vi "U6 Four 32-bit Frequency Measurements.vi"() -> ()   [LabVIEW 2021]
panel:
  out "Frequency (FIO3)":dbl format="%.2f"
  out "Period (FIO3)":dbl format="%.6f"
  out "Frequency (FIO2)":dbl format="%.2f"
  out "Period (FIO2)":dbl format="%.6f"
  in  "DeviceType":u16(ring)=1 items=["LJ_dtU3", "LJ_dtU6", "LJ_dtUE9"]
  out "Frequency (FIO1)":dbl format="%.2f"
  out "Period (FIO1)":dbl format="%.6f"
  out "Iteration":i32
  out "Frequency (FIO0)":dbl format="%.2f"
  out "Period (FIO0)":dbl format="%.6f"
  in  "error in":errorcluster
  in  "ConnectionType":u16(ring) items=["LJ_ctUSB", "LJ_ctETHERNET"]
  in  "Address":string="1"
  in  "FirstFound":bool=TRUE
  in  "stop":bool
  out "error out":errorcluster
  out "Error Message":string
  # "Each iteration, this VI measures the frequency on FIO0-FIO3 using timer mode 2 (32-bit\nperiod measurement).\n\nTested with UD V3.18 and U6 firmware V1.13."
  # "seconds"
  # "seconds"
  # "seconds"
  # "seconds"
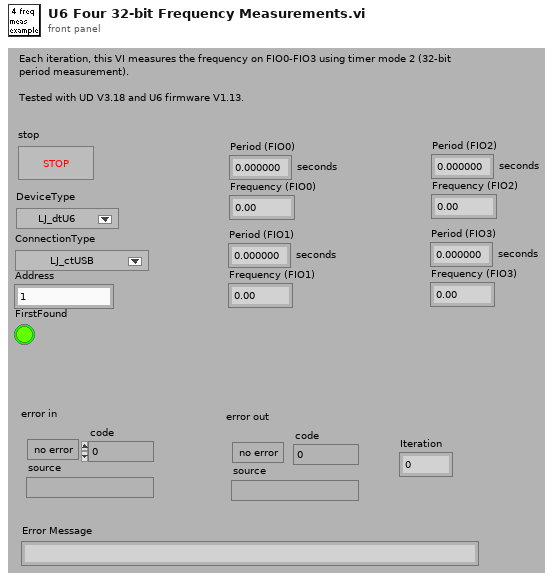
[diagram p1: front panel]
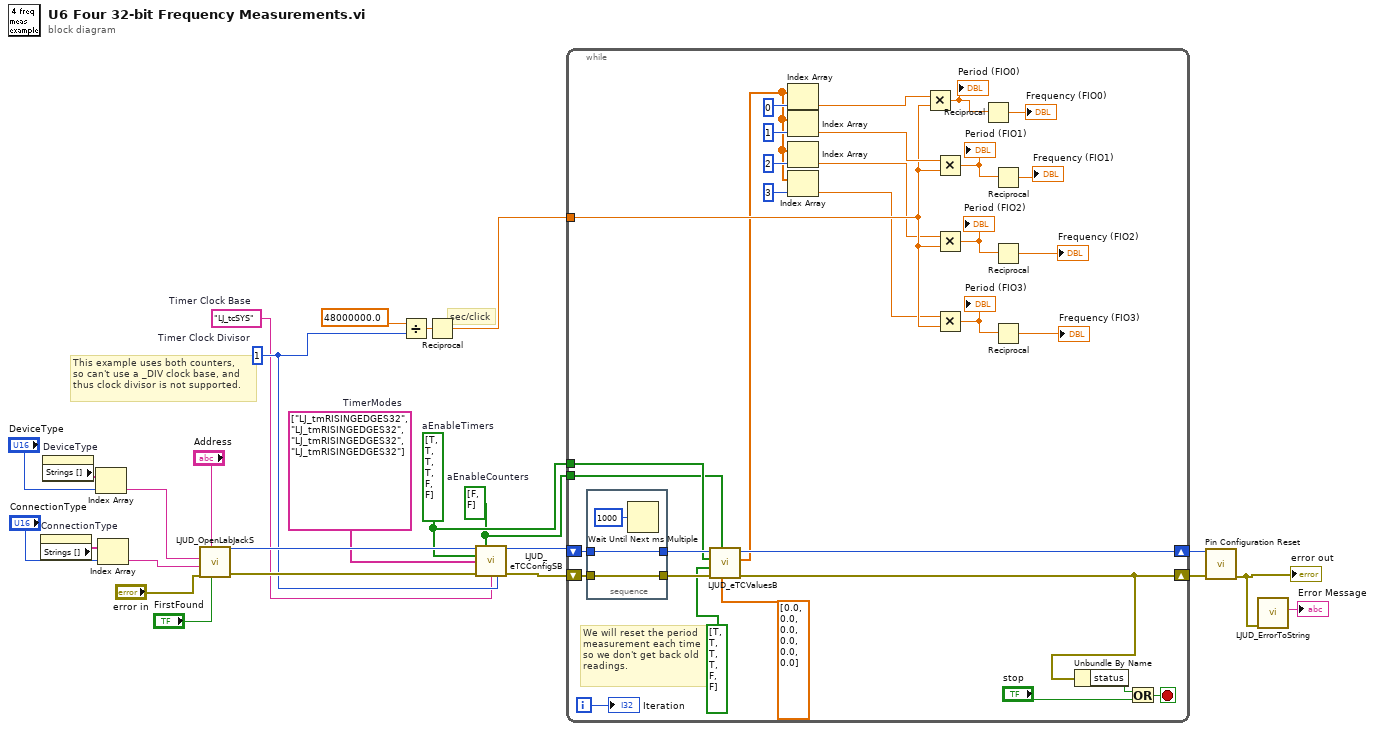
[diagram p0: block diagram]
diagram:
  w4 = bool[] [FALSE, FALSE]  # aEnableCounters
  w5 = bool[] [TRUE, TRUE, TRUE, TRUE, FALSE, FALSE]  # aEnableTimers
  w7 = 1  # Timer Clock Divisor
  w6 = "LJ_tcSYS"  # Timer Clock Base
  w8 = string[] ["LJ_tmRISINGEDGES32", "LJ_tmRISINGEDGES32", "LJ_tmRISINGEDGES32", "LJ_tmRISINGEDGES32"]  # TimerModes
  # "This example uses both counters,\nso can't use a _DIV clock base, and\nthus clock divisor is not supported."
  # "sec/click"
  n1 = property on="ConnectionType" class="Ring (strict)"() -> ("Strings []"=w17:string[])  [unwired: 2 in, 2 out]
  n2 = property on="DeviceType" class="Ring (strict)"() -> ("Strings []"=w18:string[])  [unwired: 2 in, 2 out]
  n3 = Index Array(array=w18, index="DeviceType") -> (element=w13:string)
  n4 = Index Array(array=w17, index="ConnectionType") -> (element=w14:string)
  n5 = call "LJUD_OpenLabJackS.vi"("FirstFound"="FirstFound", "Address"="Address", "error in"="error in", "ConnectionType"=w14, "DeviceType"=w13) -> ("error out"=w9:errorcluster, "Handle"=w10:i32)  [unwired: 4 in, 1 out]
  n6 = Divide(x=48000000.0, y=w7) -> (x/y=w20:dbl)
  n7 = Reciprocal(x=w20) -> (1/x=w19:dbl)
  n8 = call "LJUD_eTCConfigSB.vi"("Handle In"=w10, "aEnableCounters"=w4, "aEnableTimers"=w5, "aTimerModes"=w8, "error in"=w9, "TimerClockBase"=w6, "TimerClockDivisor"=w7) -> ("Handle Out"=w12:i32, "error out"=w11:errorcluster)  [unwired: 7 in]
  n9 = while {
    tunnel: w4 -> [w36]
    tunnel: w5 -> [w41]
    tunnel: w19 -> [w35]
    shift-left: w11 -> [w56]
    shift-right: [w44] -> w2
    shift-left: w12 -> [w57]
    shift-right: [w45] -> w3
    i -> [w48]
    stop <- w53 stop-if-true
    # "We will reset the period\nmeasurement each time\nso we don't get back old\nreadings."
    n10 = stacked-sequence {
      tunnel: [w59] -> w55
      tunnel: [w58] -> w54
      tunnel: w57 -> [w59]
      tunnel: w56 -> [w58]
      frame #0 {
        n11 = Wait Until Next ms Multiple(millisecond multiple=u32 1000) -> ()  [unwired: 1 out]
      }
    }
    n12 = call "LJUD_eTCValuesB.vi"("aTimerValues Write"=dbl[] [0.0, 0.0, 0.0, 0.0, 0.0, 0.0] ("TimerValues"), "aReadCounters"=w36, "error in"=w54, "aUpdateResetTimers"=bool[] [TRUE, TRUE, TRUE, TRUE, FALSE, FALSE] ("UpdateReset Timers"), "aReadTimers"=w41, "Handle In"=w55) -> ("error out"=w44:errorcluster, "aTimerValues Read"=w30:dbl[], "Handle Out"=w45:i32)  [unwired: 2 in, 1 out]
    n13 = Index Array(array=w30, index=0 ("Index")) -> (element=w38:dbl)
    n14 = Index Array(array=w30, index=1 ("Index")) -> (element=w37:dbl)
    n15 = Index Array(array=w30, index=2 ("Index")) -> (element=w32:dbl)
    n16 = Index Array(array=w30, index=3 ("Index")) -> (element=w31:dbl)
    n17 = Multiply(x=w38, y=w35) -> (x*y=w50:dbl)
    "Period (FIO0)" <- w50
    n18 = Multiply(x=w37, y=w35) -> (x*y=w47:dbl)
    "Period (FIO1)" <- w47
    n19 = Multiply(x=w32, y=w35) -> (x*y=w29:dbl)
    "Period (FIO2)" <- w29
    n20 = Multiply(x=w31, y=w35) -> (x*y=w27:dbl)
    "Period (FIO3)" <- w27
    n21 = Reciprocal(x=w50) -> (1/x=→"Frequency (FIO0)":dbl)
    n22 = Reciprocal(x=w47) -> (1/x=→"Frequency (FIO1)":dbl)
    n23 = Reciprocal(x=w29) -> (1/x=→"Frequency (FIO2)":dbl)
    n24 = Reciprocal(x=w27) -> (1/x=→"Frequency (FIO3)":dbl)
    n25 = Unbundle By Name(w44) -> ("status"=w52:bool)
    n26 = Or(x=w52, y="stop") -> (x .or. y?=w53:bool)
    "Iteration" <- w48
  }
  n27 = call "Pin Configuration Reset.vi"("error in"=w2, "Handle In"=w3) -> ("error out"=w1:errorcluster)  [unwired: 8 in, 1 out]
  "error out" <- w1
  n28 = call "LJUD_ErrorToString.vi"("error in"=w1) -> ("String"=→"Error Message":string)  [unwired: 10 in]
